vi "TDS Waveform Output Write.vi"(6 "Waveform Settings":T1={"Frequency"=0.0, "Amplitude"=0.0, "DC Offset"=0.0, "Duty Cycle"=-1.0, "Number of Samples"=-1, "Sample Rate"=-1}, 8 "error in (no error)":errorcluster, 9 "Waveform Type":string(combo), 10 "Signal InstConfig":string, 11 "Address":string) -> (0 "error out":errorcluster)   [LabVIEW 2025, in "Interface Functions.lvlib"]
uses:
  Interface Functions.lvlib
panel:
  # "Waveform Output Write"
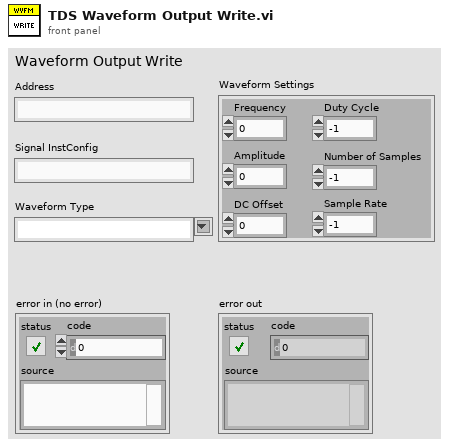
[diagram p1: front panel]
types:
  T1 = cluster{"Frequency":dbl, "Amplitude":dbl, "DC Offset":dbl, "Duty Cycle":dbl, "Number of Samples":i32, "Sample Rate":i32}
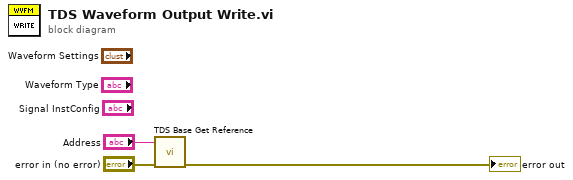
[diagram p0: block diagram]
diagram:
  n1 = call "TDS Base Get Reference.vi"("error in (no error)"="error in (no error)", "Address"="Address") -> ("error out"=→"error out":errorcluster)  [unwired: 8 in, 1 out]
